vi "Main.vi"() -> ()   [LabVIEW 2015]
doc: "The myRIO Project template acquires acceleration data from the onboard accelerometer and displays the changes of acceleration values in a waveform chart."
uses:
  <vilib>/myRIO/Instrument Drivers/Onboard IO/DIO/typedefs/DIO Reference.ctl
  <vilib>/myRIO/Common/Instrument Driver Framework/Utilities/typedefs/myRIO Generic Hardware Reference.ctl
  <vilib>/myRIO/Common/Instrument Driver Framework/Utilities/typedefs/Hardware Version Enum.ctl
  <vilib>/myRIO/Common/Instrument Driver Framework/Utilities/typedefs/myRIO v1.0 Reference.ctl
  <vilib>/myRIO/Common/Instrument Driver Framework/Utilities/typedefs/Generic FPGA Reference.ctl
  <vilib>/myRIO/Common/Instrument Driver Framework/myRIO v1.0/DIO/typedefs/DIO Channels List.ctl
  <vilib>/myRIO/Common/Instrument Driver Framework/myRIO v1.0/DIO/typedefs/DIO Channels Enum.ctl
  <vilib>/userdefined/High Color/nirio_resource_hc.ctl
  <vilib>/myRIO/Instrument Drivers/Onboard IO/PWM/typedefs/PWM Reference.ctl
  <vilib>/myRIO/Common/Instrument Driver Framework/myRIO v1.0/PWM/typedefs/PWM Channels Enum.ctl
  <vilib>/myRIO/Instrument Drivers/Onboard IO/PWM/typedefs/PWM Configuration.ctl
  <vilib>/myRIO/Instrument Drivers/Onboard Devices/Accelerometer/typedefs/Accelerometer Reference.ctl
  <vilib>/myRIO/Common/Instrument Driver Framework/myRIO v1.0/Accelerometer/typedefs/Accelerometer Channels List.ctl
  <vilib>/myRIO/Common/Instrument Driver Framework/myRIO v1.0/Accelerometer/typedefs/Accelerometer Channels Enum.ctl
  <vilib>/myRIO/Common/Instrument Driver Framework/Utilities/vis/Is FPGA Ref Available.vi
  <vilib>/myRIO/Common/Instrument Driver Framework/myRIO v1.0/DIO/vis/myRIO v1.1 Open DIO.vi
  <vilib>/myRIO/Instrument Drivers/Onboard IO/DIO/vis/Write.vi
  <vilib>/myRIO/Common/Instrument Driver Framework/myRIO v1.0/PWM/vis/myRIO v1.1 Open PWM.vi
  <vilib>/myRIO/Instrument Drivers/Onboard IO/PWM/vis/Set Duty Cycle and Frequency.vi
  <vilib>/myRIO/Common/Instrument Driver Framework/myRIO v1.0/Accelerometer/vis/myRIO v1.1 Open Accelerometer.vi
  <vilib>/myRIO/Instrument Drivers/Onboard Devices/Accelerometer/vis/Read.vi
  <vilib>/myRIO/Common/Instrument Driver Framework/Utilities/vis/Validate Channels.vi
  <vilib>/myRIO/Common/Instrument Driver Framework/myRIO v1.0/DIO/vis/myRIO v1.0 Reserve DIO.vi
  <vilib>/myRIO/Common/Instrument Driver Framework/myRIO v1.0/PWM/vis/myRIO v1.0 Reserve PWM.vi
  <vilib>/myRIO/Common/Instrument Driver Framework/myRIO v1.0/Accelerometer/vis/myRIO v1.0 Reserve Accelerometer.vi
  <vilib>/myRIO/Common/Instrument Driver Framework/myRIO v1.0/UART/vis/myRIO v1.0 Close UART.vi
  <vilib>/myRIO/Common/Instrument Driver Framework/myRIO v1.0/Resource Manager/vis/myRIO v1.0 Reserve Channel List.vi
  <vilib>/myRIO/Common/Instrument Driver Framework/myRIO v1.0/DIO/vis/myRIO v1.0 Build MUX Configuration DIO.vi
  <vilib>/myRIO/Common/Instrument Driver Framework/myRIO v1.0/PWM/vis/myRIO v1.0 Build MUX Configuration PWM.vi
  <vilib>/myRIO/Common/Instrument Driver Framework/myRIO v1.0/Accelerometer/vis/myRIO v1.0 Build MUX Configuration Accelerometer.vi
  <vilib>/myRIO/Common/Instrument Driver Framework/myRIO v1.0/Resource Manager/vis/myRIO v1.0 Reserve Channel.vi
  <vilib>/myRIO/Common/Instrument Driver Framework/myRIO v1.0/Resource Manager/vis/myRIO v1.0 Unreserve Channel.vi
  <vilib>/myRIO/Common/Instrument Driver Framework/myRIO v1.0/Resource Manager/vis/myRIO v1.0 Create Configuration List.vi
  <vilib>/myRIO/Common/Instrument Driver Framework/myRIO v1.0/Resource Manager/vis/myRIO v1.0 Build Mutex Name.vi
  <vilib>/Utility/VariantDataType/GetNumericInfo.vi
  <vilib>/Utility/error.llb/Error Cluster From Error Code.vi
  <vilib>/myRIO/Common/Instrument Driver Framework/myRIO v1.0/myRIO v1.1 Open.vi
  <vilib>/myRIO/Common/Instrument Driver Framework/Utilities/vis/IO Manager.vi
  <vilib>/myRIO/Common/Instrument Driver Framework/Utilities/vis/Configuration Manager.vi
  <vilib>/myRIO/Common/Instrument Driver Framework/myRIO v1.0/Resource Manager/vis/myRIO v1.0 Configure IO.vi
  <vilib>/myRIO/Common/Instrument Driver Framework/myRIO v1.0/myRIO v1.0 Close.vi
  <vilib>/myRIO/Common/Instrument Driver Framework/myRIO v1.0/PWM/vis/myRIO v1.0 Write PWM.vi
  <vilib>/myRIO/Common/Instrument Driver Framework/myRIO v1.0/DIO/vis/myRIO v1.0 Write DIO.vi
  <vilib>/myRIO/Common/Instrument Driver Framework/myRIO v1.0/Accelerometer/vis/myRIO v1.0 Get Scaling Constant Accelerometer.vi
  <vilib>/myRIO/Common/Instrument Driver Framework/myRIO v1.0/Accelerometer/vis/myRIO v1.0 Read Accelerometer.vi
  <vilib>/myRIO/Common/Instrument Driver Framework/Utilities/vis/FPGA Ref Manager.vi
  <vilib>/myRIO/Common/Instrument Driver Framework/myRIO v1.0/myRIO v1.0 Reset FPGA.vi
  <vilib>/myRIO/Common/Instrument Driver Framework/myRIO v1.0/IRQ/vis/myRIO v1.0 IRQ Info FGV.vi
  <vilib>/myRIO/Common/Instrument Driver Framework/myRIO v1.0/IRQ/vis/myRIO v1.0 Timer IRQ Info FGV.vi
  <vilib>/myRIO/Common/Instrument Driver Framework/myRIO v1.0/IRQ/vis/myRIO v1.0 ISR Agent.vi
  <vilib>/myRIO/Express VI/Onboard IO/PWM/PWM Express VI.xnode
  <vilib>/myRIO/Instrument Drivers/Onboard IO/PWM/vis/myRIO PWM Open.xnode
  <vilib>/myRIO/Express VI/Onboard IO/DO/DO Express VI.xnode
  <vilib>/myRIO/Instrument Drivers/Onboard IO/DIO/vis/myRIO DIO Open.xnode
  <vilib>/myRIO/Express VI/Onboard Devices/Accelerometer/Accelerometer Express VI.xnode
  <vilib>/myRIO/Instrument Drivers/Onboard Devices/Accelerometer/vis/myRIO Accelerometer Open.xnode
  <vilib>/myRIO/Instrument Drivers/Utilities/Utilities.lvlib
  <vilib>/myRIO/Instrument Drivers/Onboard Devices/Accelerometer/Accelerometer.lvlib
  <vilib>/myRIO/Instrument Drivers/Onboard IO/PWM/PWM.lvlib
  <vilib>/myRIO/Instrument Drivers/Onboard IO/DIO/DIO.lvlib
panel:
  in  "right dist":dbl
  in  "left dist":dbl
  out "波形图表 2":dbl(graph)
  in  "right":bool
  in  "left":bool
  out "Acceleration":T1(graph)
  out "error out":errorcluster
  in  "Stop":bool
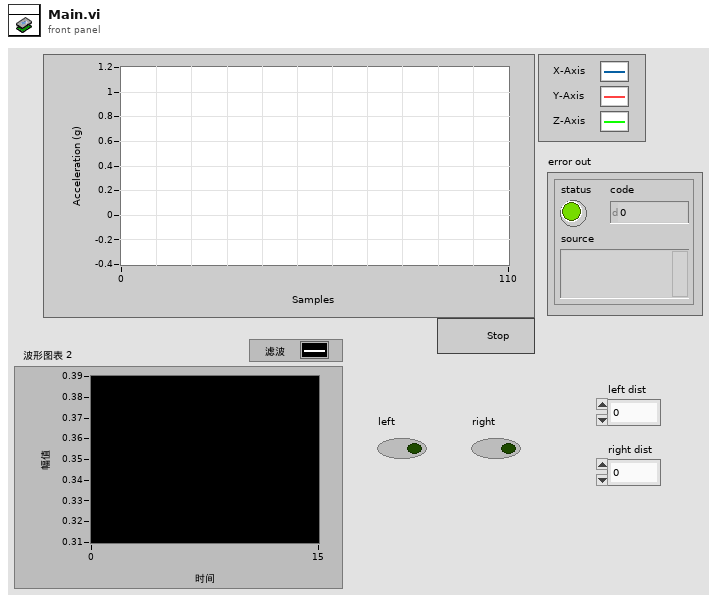
[diagram p1: front panel]
types:
  T1 = cluster{"X-Axis":dbl, "Y-Axis":dbl, "Z-Axis":dbl}
  T2 = typedef "DIO.lvlib/DIO Reference.ctl" = cluster{"myRIO Reference":T3, "DIO Channels List":T7}
  T3 = typedef "myRIO Generic Hardware Reference.ctl" = cluster{"myRIO Model":T4, "myRIO Hardware Reference":T5}
  T4 = typedef "Hardware Version Enum.ctl" = enum16{"Unknown", "myRIO-1900", "myRIO-1950", "roboRIO"}
  T5 = typedef "myRIO v1.0 Reference.ctl" = cluster{"Generic FPGA Reference":T6, "Allow multiple opens":bool}
  T6 = typedef "Generic FPGA Reference.ctl" = refnum<k20>
  T7 = typedef "DIO Channels List.ctl" = T8[]
  T8 = typedef "DIO Channels Enum.ctl" = enum16{"Not Connected", "C/DIO0", "C/DIO1", "C/DIO2", "C/DIO3", "C/DIO4", "C/DIO5", "C/DIO6", "C/DIO7", "A/DIO0", "A/DIO1", "A/DIO2", "A/DIO3", "A/DIO4", "A/DIO5", "A/DIO6", "A/DIO7", "A/DIO8", "A/DIO9", "A/DIO10", "A/DIO11", "A/DIO12", "A/DIO13", "A/DIO14", "A/DIO15", "B/DIO0", "B/DIO1", "B/DIO2", "B/DIO3", "B/DIO4", "B/DIO5", "B/DIO6", "B/DIO7", "B/DIO8", "B/DIO9", "B/DIO10", "B/DIO11", "B/DIO12", "B/DIO13", "B/DIO14", "B/DIO15", "LED0", "LED1", "LED2", "LED3", "Button0", "DIO/DIO0", "DIO/DIO1", "DIO/DIO2", "DIO/DIO3", "DIO/DIO4", "DIO/DIO5", "DIO/DIO6", "DIO/DIO7", "DIO/DIO8", "DIO/DIO9", "SPI/CS0", "SPI/CS1", "SPI/CS2", "SPI/CS3", "LED RADIO (Green)", "LED RADIO (Red)", "LED COMM (Green)", "LED COMM (Red)", "LED MODE (Green)", "LED MODE (Red)"}
  T9 = typedef "nirio_resource_hc.ctl" = tag
  T10 = typedef "PWM.lvlib/PWM Reference.ctl" = cluster{"myRIO Reference":T3, "PWM Channels Enum":T11, "PWM Configuration":T12}
  T11 = typedef "PWM Channels Enum.ctl" = enum16{"Not Connected", "C/PWM0", "C/PWM1", "A/PWM0", "A/PWM1", "A/PWM2", "B/PWM0", "B/PWM1", "B/PWM2", "PWM/PWM0", "PWM/PWM1", "PWM/PWM2", "PWM/PWM3", "PWM/PWM4", "PWM/PWM5", "PWM/PWM6", "PWM/PWM7", "PWM/PWM8", "PWM/PWM9"}
  T12 = typedef "PWM.lvlib/PWM Configuration.ctl" = cluster{"Frequency":dbl, "Duty Cycle":dbl}
  T13 = typedef "Accelerometer.lvlib/Accelerometer Reference.ctl" = cluster{"myRIO Reference":T3, "Accelerometer Channels List":T14, "LSB Weight":dbl}
  T14 = typedef "Accelerometer Channels List.ctl" = T15[]
  T15 = typedef "Accelerometer Channels Enum.ctl" = enum16{"Not Connected", "X-Axis", "Y-Axis", "Z-Axis"}
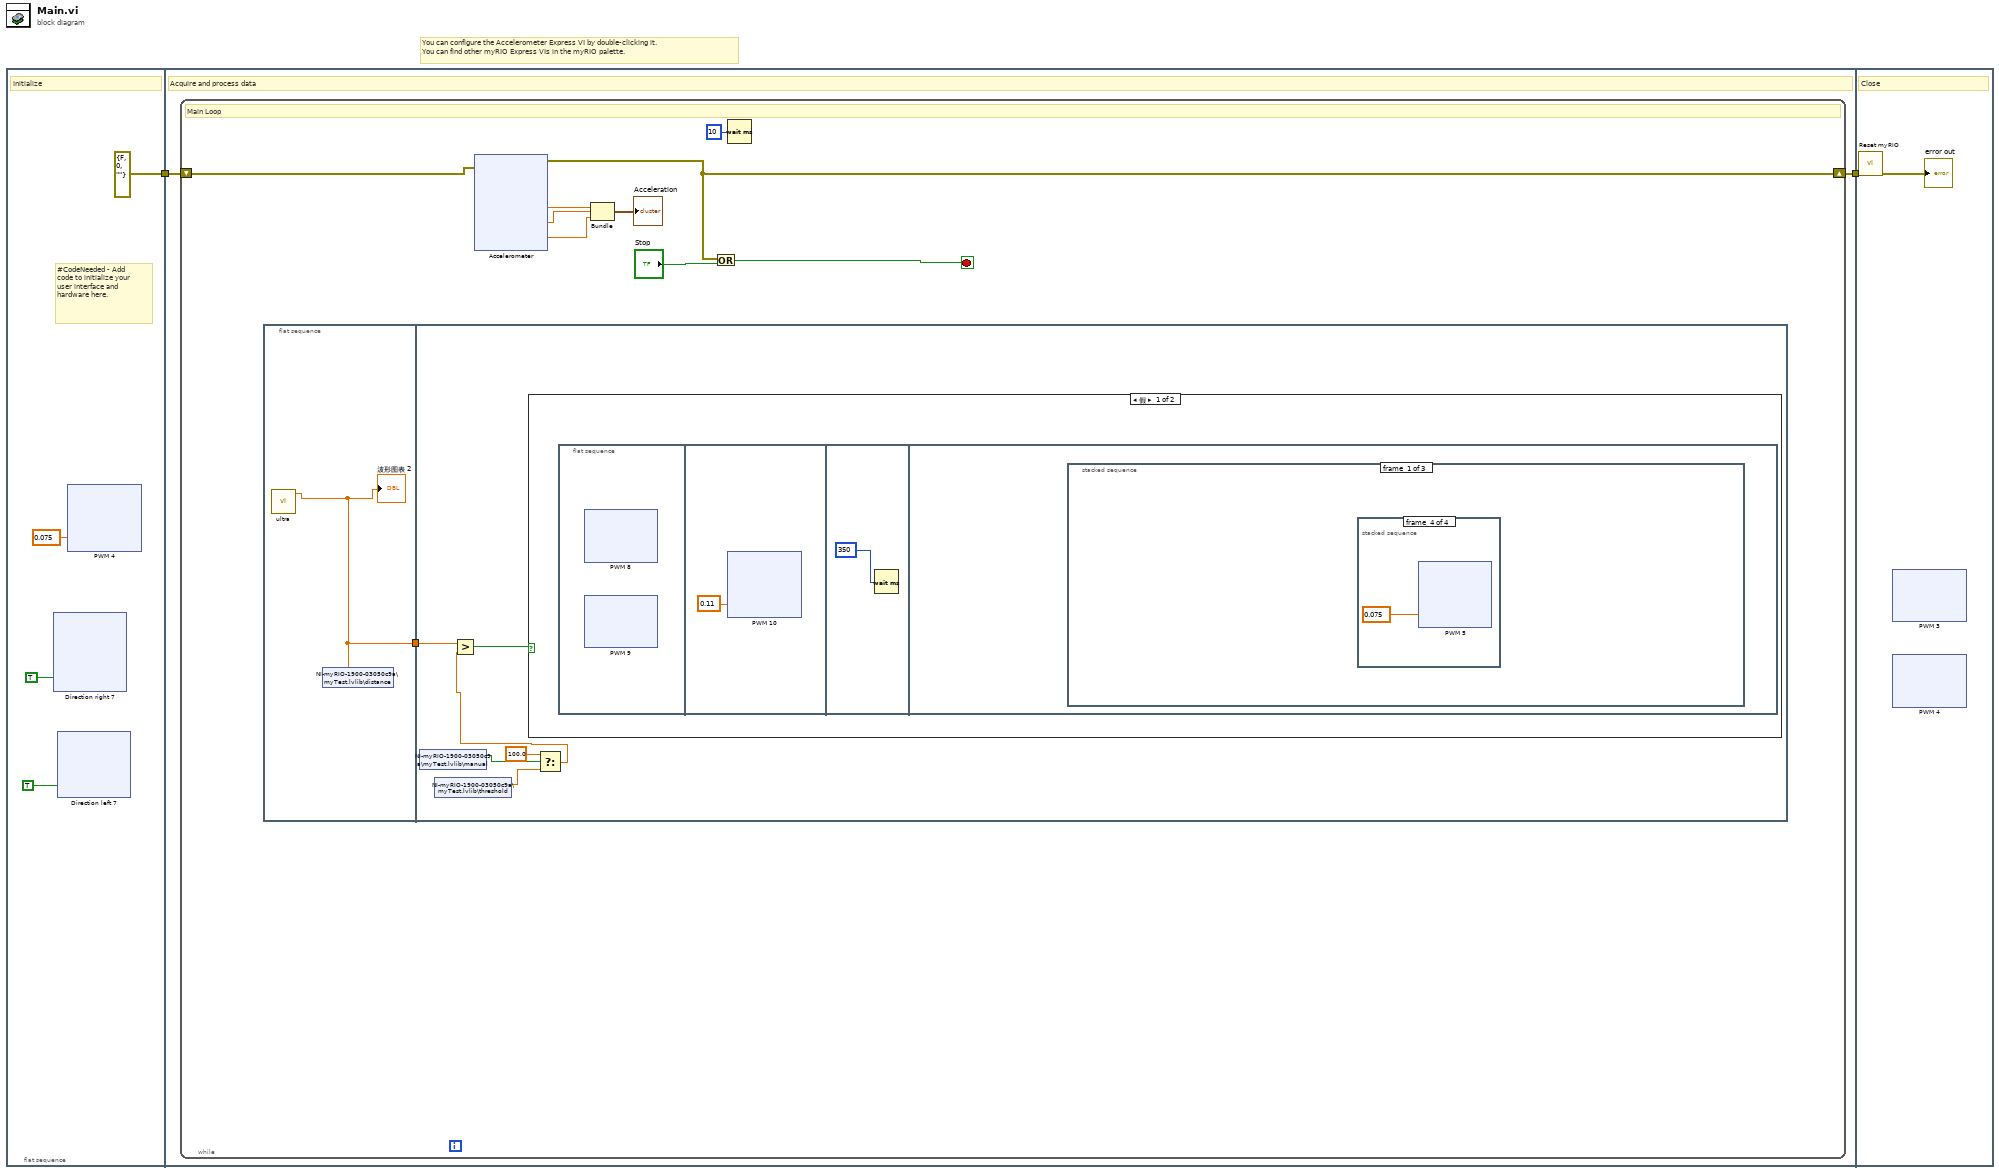
[diagram p0: block diagram]
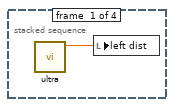
[diagram p2: hidden frame]
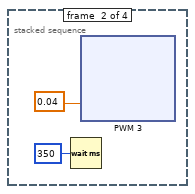
[diagram p3: hidden frame]
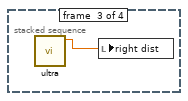
[diagram p4: hidden frame]
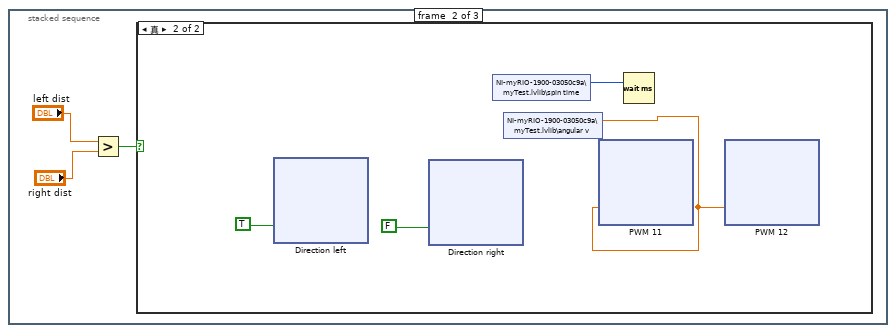
[diagram p5: hidden frame]
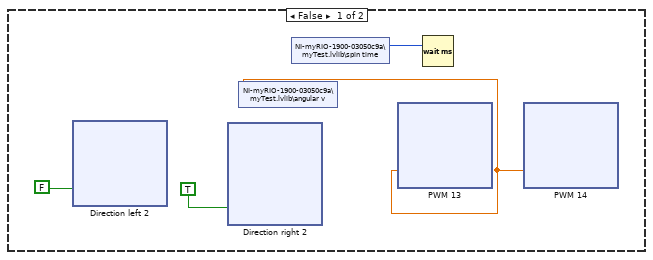
[diagram p6: hidden frame]
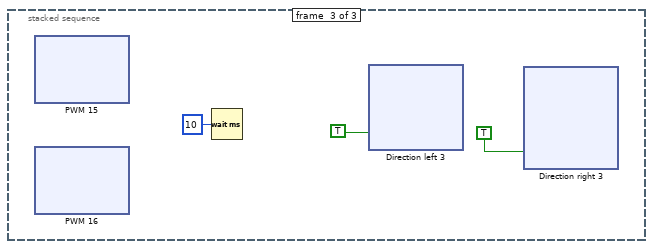
[diagram p7: hidden frame]
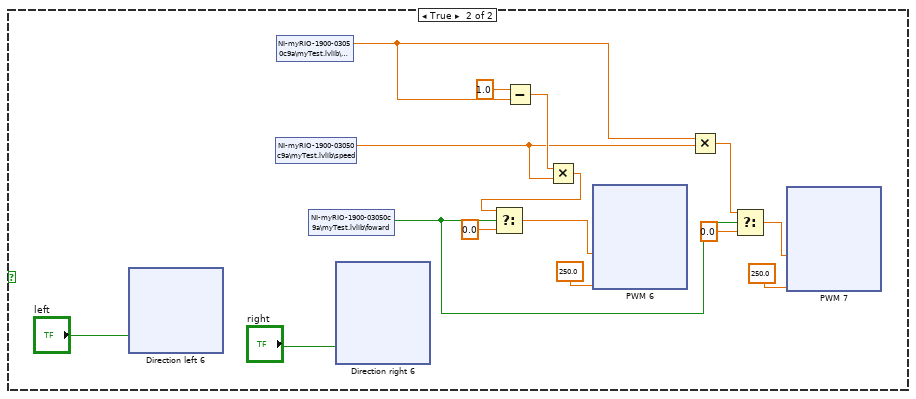
[diagram p8: hidden frame]
diagram:
  # "You can configure the Accelerometer Express VI by double-clicking it.\nYou can find other myRIO Express VIs in the myRIO palette."
  n1 = flat-sequence {
    tunnel: [errorcluster {"status"=FALSE, "code"=0, "source"=""} ("error in (no error)")] -> w2
    tunnel: w2 -> [w113]
    tunnel: [w112] -> w1
    tunnel: w1 -> [w942]
    frame #0 {
      # "#CodeNeeded - Add code to initialize your user interface and hardware here."
      # "Initialize"
      n2 = xnode "Direction right 7"("A/DIO3 (Pin 17)"=TRUE) -> ()  [unwired: 1 in, 1 out]
      n3 = xnode "Direction left 7"("B/DIO3 (Pin 17)"=TRUE) -> ()  [unwired: 1 in, 1 out]
      n4 = xnode "PWM 4"("Duty Cycle"=0.075) -> ()  [unwired: 1 in, 1 out]
    }
    frame #1 {
      # "Acquire and process data"
      n5 = while {
        shift-right: [w119] -> w112
        shift-left: w113 -> [w116]
        stop <- w122 stop-if-true
        # "Main Loop"
        n6 = flat-sequence {
          tunnel: [w124] -> w115
          tunnel: w115 -> [w129]
          frame #0 {
            n7 = call "ultra.vi"() -> ("数值"=w124:dbl)  [unwired: 11 in]
            "波形图表 2" <- w124
            n8 = shared-variable "NI-myRIO-1900-03050c9a\\myTest.lvlib\\distance"(w124) -> ()  [unwired: 1 in, 1 out]
          }
          frame #1 {
            n9 = shared-variable "NI-myRIO-1900-03050c9a\\myTest.lvlib\\manual"() -> (w128:bool)  [unwired: 1 in, 1 out]
            n10 = shared-variable "NI-myRIO-1900-03050c9a\\myTest.lvlib\\threshold"() -> (w126:dbl)  [unwired: 1 in, 1 out]
            n11 = Select(t=100.0, s=w128, f=w126) -> (s? t:f=w125:dbl)
            n12 = Greater?(x=w129, y=w125) -> (0:w130:bool)
            n13 = case shown="假" w130 {
              frame False {
                n14 = flat-sequence {
                  frame #0 {
                    n15 = xnode "PWM 8"() -> ()  [unwired: 1 in, 1 out]
                    n16 = xnode "PWM 9"() -> ()  [unwired: 1 in, 1 out]
                  }
                  frame #1 {
                    n17 = xnode "PWM 10"("Duty Cycle"=0.11) -> ()  [unwired: 1 in, 1 out]
                  }
                  frame #2 {
                    n18 = Wait (ms)(milliseconds to wait=350) -> ()  [unwired: 1 out]
                  }
                  frame #3 {
                    n19 = stacked-sequence {
                      frame #0 {
                        n20 = stacked-sequence {
                          frame #0 {
                            n21 = call "ultra.vi"() -> ("数值"=w238:dbl)  [unwired: 11 in]
                            n22 = local write "left dist"(w238) -> ()
                          }
                          frame #1 {
                            n23 = Wait (ms)(milliseconds to wait=u32 350 ("等待时间（毫秒）")) -> ()  [unwired: 1 out]
                            n24 = xnode "PWM 3"("Duty Cycle"=0.04) -> ()  [unwired: 1 in, 1 out]
                          }
                          frame #2 {
                            n25 = call "ultra.vi"() -> ("数值"=w276:dbl)  [unwired: 11 in]
                            n26 = local write "right dist"(w276) -> ()
                          }
                          frame #3 {
                            n27 = xnode "PWM 5"("Duty Cycle"=0.075) -> ()  [unwired: 1 in, 1 out]
                          }
                        }
                      }
                      frame #1 {
                        n28 = Greater?(x="left dist", y="right dist") -> (0:w313:bool)
                        n29 = case shown="真" w313 {
                          frame False {
                            n30 = xnode "Direction left 2"("B/DIO3 (Pin 17)"=FALSE) -> ()  [unwired: 1 in, 1 out]
                            n31 = xnode "Direction right 2"("A/DIO3 (Pin 17)"=TRUE) -> ()  [unwired: 1 in, 1 out]
                            n32 = shared-variable "NI-myRIO-1900-03050c9a\\myTest.lvlib\\angular v"() -> (w316:dbl)  [unwired: 1 in, 1 out]
                            n33 = shared-variable "NI-myRIO-1900-03050c9a\\myTest.lvlib\\spin time"() -> (w319:u32)  [unwired: 1 in, 1 out]
                            n34 = xnode "PWM 13"("Duty Cycle"=w316) -> ()  [unwired: 1 in, 1 out]
                            n35 = Wait (ms)(milliseconds to wait=w319) -> ()  [unwired: 1 out]
                            n36 = xnode "PWM 14"("Duty Cycle"=w316) -> ()  [unwired: 1 in, 1 out]
                          }
                          frame True {
                            n37 = xnode "Direction left"("B/DIO3 (Pin 17)"=TRUE) -> ()  [unwired: 1 in, 1 out]
                            n38 = xnode "Direction right"("A/DIO3 (Pin 17)"=FALSE) -> ()  [unwired: 1 in, 1 out]
                            n39 = shared-variable "NI-myRIO-1900-03050c9a\\myTest.lvlib\\spin time"() -> (w463:u32)  [unwired: 1 in, 1 out]
                            n40 = shared-variable "NI-myRIO-1900-03050c9a\\myTest.lvlib\\angular v"() -> (w460:dbl)  [unwired: 1 in, 1 out]
                            n41 = xnode "PWM 11"("Duty Cycle"=w460) -> ()  [unwired: 1 in, 1 out]
                            n42 = Wait (ms)(milliseconds to wait=w463) -> ()  [unwired: 1 out]
                            n43 = xnode "PWM 12"("Duty Cycle"=w460) -> ()  [unwired: 1 in, 1 out]
                          }
                        }
                      }
                      frame #2 {
                        n44 = xnode "PWM 15"() -> ()  [unwired: 1 in, 1 out]
                        n45 = xnode "PWM 16"() -> ()  [unwired: 1 in, 1 out]
                        n46 = Wait (ms)(milliseconds to wait=u32 10 ("等待时间（毫秒）")) -> ()  [unwired: 1 out]
                        n47 = xnode "Direction left 3"("B/DIO3 (Pin 17)"=TRUE) -> ()  [unwired: 1 in, 1 out]
                        n48 = xnode "Direction right 3"("A/DIO3 (Pin 17)"=TRUE) -> ()  [unwired: 1 in, 1 out]
                      }
                    }
                  }
                }
              }
              frame True {
                n49 = xnode "Direction left 6"("B/DIO3 (Pin 17)"="left") -> ()  [unwired: 1 in, 1 out]
                n50 = shared-variable "NI-myRIO-1900-03050c9a\\myTest.lvlib\\speed"() -> (w758:dbl)  [unwired: 1 in, 1 out]
                n51 = shared-variable "NI-myRIO-1900-03050c9a\\myTest.lvlib\\angle"() -> (w761:dbl)  [unwired: 1 in, 1 out]
                n52 = shared-variable "NI-myRIO-1900-03050c9a\\myTest.lvlib\\foward"() -> (w757:bool)  [unwired: 1 in, 1 out]
                n53 = xnode "Direction right 6"("A/DIO3 (Pin 17)"="right") -> ()  [unwired: 1 in, 1 out]
                n54 = Subtract(x=1.0, y=w761) -> (x-y=w759:dbl)
                n55 = Multiply(x=w759, y=w758) -> (x*y=w753:dbl)
                n56 = Select(t=w753, s=w757, f=0.0) -> (s? t:f=w752:dbl)
                n57 = xnode "PWM 6"("Duty Cycle"=w752, "Frequency [Hz]"=250.0) -> ()  [unwired: 1 in, 1 out]
                n58 = Multiply(x=w761, y=w758) -> (x*y=w756:dbl)
                n59 = Select(t=w756, s=w757, f=0.0) -> (s? t:f=w751:dbl)
                n60 = xnode "PWM 7"("Duty Cycle"=w751, "Frequency [Hz]"=250.0) -> ()  [unwired: 1 in, 1 out]
              }
            }
          }
        }
        n61 = xnode "Accelerometer"("error in (no error)"=w116) -> ("X-Axis"=w114:dbl, "Y-Axis"=w117:dbl, "Z-Axis"=w118:dbl, "error out"=w119:errorcluster)
        n62 = Bundle("X-Axis"=w114, "Y-Axis"=w117, "Z-Axis"=w118) -> (→"Acceleration":T1)  [unwired: 1 in]
        n63 = Or(x=w119, y="Stop") -> (x .or. y?=w122:bool)
        n64 = Wait (ms)(milliseconds to wait=u32 10) -> ()  [unwired: 1 out]
      }
    }
    frame #2 {
      # "Close"
      n65 = call <vilib>:"Reset myRIO.vi"("error in (no error)"=w942) -> ("error out"=→"error out":errorcluster)  [unwired: 10 in]
      n66 = xnode "PWM 3"() -> ()  [unwired: 1 in, 1 out]
      n67 = xnode "PWM 4"() -> ()  [unwired: 1 in, 1 out]
    }
  }
